vi "Result_Test.vi"(8 "error in (no error)":errorcluster caption="entrée d'erreur (pas d'erreur)", 11 "Get_Voltage en entrée":refnum<class "Zigbee_Send_Msg_Model_Identifier.lvclass">) -> (0 "error out":errorcluster caption="sortie d'erreur", 3 "Get_Voltage en sortie":refnum<class "Zigbee_Send_Msg_Model_Identifier.lvclass">)   [LabVIEW 2020, in "Library Test.lvlib" / "Zigbee_Send_Msg_Model_Identifier.lvclass"]
uses:
  Zigbee_Send_Msg_Model_Identifier.lvclass
  C:/Users/ngarcin/OneDrive - Altyor/Standard TB/Class/Test/Zigbee_Send_Msg/Zigbee_Send_Msg.lvclass
  C:/Users/ngarcin/OneDrive - Altyor/Standard TB/Class/Test/Test (Default)/Test (Default).lvclass
  Zigbee_Send_Msg/Zigbee_Send_Msg.lvclass
  Zigbee_Send_Msg_Model_Identifier.lvclass/Zigbee_Send_Msg_Model_Identifier.ctl
  Commun VI/Library Commun.lvlib
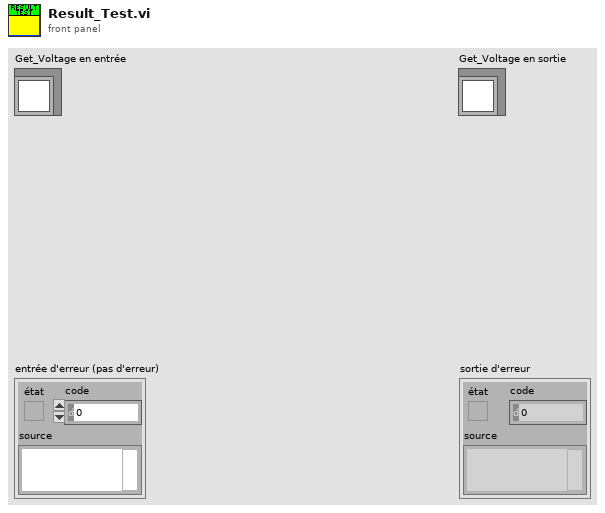
[diagram p1: front panel]
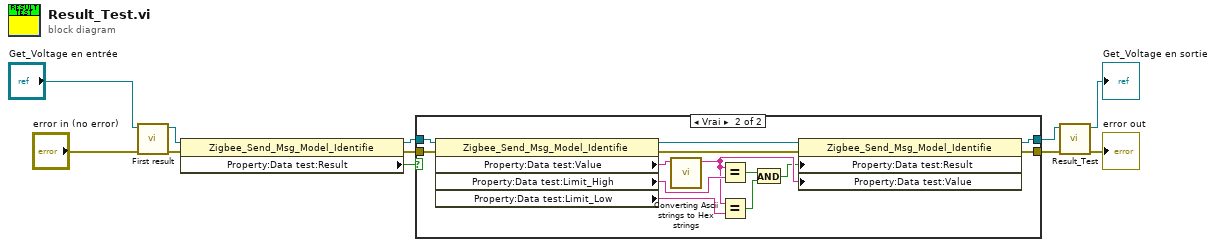
[diagram p0: block diagram]
diagram:
  n1 = call "First result.vi"("entrée d'erreur (pas d'erreur)"="error in (no error)", "Zigbee_Send_Msg en entrée"="Get_Voltage en entrée") -> ("sortie d'erreur"=w3:errorcluster, "Zigbee_Send_Msg en sortie"=w1:refnum<class "Zigbee_Send_Msg_Model_Identifier.lvclass">)  [unwired: 7 in, 1 out]
  n2 = property class="Zigbee_Send_Msg_Model_Identifie"(reference=w1, error in=w3) -> (reference out=w9:refnum<class "Zigbee_Send_Msg_Model_Identifier.lvclass">, error out=w10:errorcluster, "Property:Data test:Result"=w11:bool)
  n3 = case shown="Vrai" w11 {
    tunnel: w10 -> [w12 w25]
    tunnel: [w12 w24] -> w7
    tunnel: [w13 w23] -> w8
    tunnel: w9 -> [w13 w22]
    frame False {
    }
    frame True {
      n4 = property class="Zigbee_Send_Msg_Model_Identifie"(reference=w22, error in=w25) -> (reference out=w26:refnum<class "Zigbee_Send_Msg_Model_Identifier.lvclass">, error out=w14:errorcluster, "Property:Data test:Value"=w21:string, "Property:Data test:Limit_High"=w20:string, "Property:Data test:Limit_Low"=w19:string)
      n5 = call "Converting Ascii strings to Hex strings.vi"("result string"=w21) -> ("Chaîne"=w18:string)  [unwired: 10 in]
      n6 = Equal?(x=w18, y=w20) -> (x = y?=w16:bool)
      n7 = Equal?(x=w18, y=w19) -> (x = y?=w17:bool)
      n8 = And(x=w16, y=w17) -> (x .and. y?=w15:bool)
      n9 = property class="Zigbee_Send_Msg_Model_Identifie"(reference=w26, error in=w14, "Property:Data test:Result"=w15, "Property:Data test:Value"=w18) -> (reference out=w23:refnum<class "Zigbee_Send_Msg_Model_Identifier.lvclass">, error out=w24:errorcluster)
    }
  }
  n10 = call-parent "Result_Test.vi"("error in (no error)"=w7, "Get_Voltage en entrée"=w8) -> ("error out"=→"error out":errorcluster, "Get_Voltage en sortie"=→"Get_Voltage en sortie":refnum<class "Zigbee_Send_Msg_Model_Identifier.lvclass">)  [unwired: 8 in]
